vi "LSMcontroller_v65_updatedsealtest.vi"() -> ()   [LabVIEW 2015] (continued)
                    n3079 = property on="save\ndata" class="Bool (strict)"("Value"=TRUE ("save\ndata")) -> ()  [unwired: 2 in, 2 out]
                    n3080 = property on="# of frames" class="DigNum (strict)"("DisabledEnum"=T7."Enabled" ("Disabled")) -> ()  [unwired: 2 in, 2 out]
                  }
                }
              }
              frame #1 {
                n3081 = local read "finite samples"() -> (w6307:bool)
                n3082 = local read "continuous"() -> (w6306:bool)
                n3083 = local read "wavdet"() -> (w6305:bool)
                n3084 = call "2pparameters.vi"("command"="get") -> ("params out"=w6301:T10)  [unwired: 1 in]
                n3085 = Bundle By Name(cluster=w6301, "finite"=w6307, "cont"=w6306, "wavdet"=w6305) -> (w6304:T10)
                n3086 = call "2pparameters.vi"("Params in"=w6304, "command"="set") -> ()  [unwired: 1 out]
              }
            }
          }
          event "continuous": Value Change {
            n3087 = event-data() -> ("NewVal"=w6308:bool)  [unwired: 1 in]
            n3088 = flat-sequence {
              tunnel: w6308 -> [w6309]
              frame #0 {
                n3089 = case shown="True" w6309 {
                  frame False {
                    n3090 = property on="finite samples" class="Bool (strict)"("Value"=TRUE ("finite samples for recording")) -> ()  [unwired: 2 in, 2 out]
                    n3091 = property on="save\ndata" class="Bool (strict)"("Value"=TRUE ("save\ndata")) -> ()  [unwired: 2 in, 2 out]
                    n3092 = property on="wavdet" class="Bool (strict)"("Value"=FALSE ("wavdet")) -> ()  [unwired: 2 in, 2 out]
                    n3093 = local write "Save tab"(enum32{"withsave", "withoutsave"}."withsave" ("Save tab")) -> ()
                    n3094 = property on="# of frames" class="DigNum (strict)"("DisabledEnum"=T7."Enabled" ("Disabled")) -> ()  [unwired: 2 in, 2 out]
                    n3095 = property on="save\ndata" class="Bool (strict)"("DisabledEnum"=T7."Enabled" ("Disabled")) -> ()  [unwired: 2 in, 2 out]
                  }
                  frame True {
                    w6316 = FALSE ("finite samples for recording")
                    n3096 = property on="finite samples" class="Bool (strict)"("Value"=w6316) -> ()  [unwired: 2 in, 2 out]
                    n3097 = property on="wavdet" class="Bool (strict)"("Value"=w6316) -> ()  [unwired: 2 in, 2 out]
                    n3098 = property on="save\ndata" class="Bool (strict)"("Value"=w6316) -> ()  [unwired: 2 in, 2 out]
                    n3099 = local write "Save tab"(enum32{"withsave", "withoutsave"}."withsave" ("Save tab")) -> ()
                    n3100 = property on="# of frames" class="DigNum (strict)"("DisabledEnum"=T7."Disabled and Grayed Out" ("Disabled")) -> ()  [unwired: 2 in, 2 out]
                    n3101 = property on="save\ndata" class="Bool (strict)"("DisabledEnum"=T7."Disabled and Grayed Out" ("Disabled")) -> ()  [unwired: 2 in, 2 out]
                  }
                }
              }
              frame #1 {
                n3102 = local read "finite samples"() -> (w6326:bool)
                n3103 = local read "continuous"() -> (w6325:bool)
                n3104 = local read "wavdet"() -> (w6324:bool)
                n3105 = call "2pparameters.vi"("command"="get") -> ("params out"=w6320:T10)  [unwired: 1 in]
                n3106 = Bundle By Name(cluster=w6320, "finite"=w6326, "cont"=w6325, "wavdet"=w6324) -> (w6323:T10)
                n3107 = call "2pparameters.vi"("Params in"=w6323, "command"="set") -> ()  [unwired: 1 out]
              }
            }
          }
          event "wavdet": Value Change {
            n3108 = event-data() -> ("NewVal"=w6327:bool)  [unwired: 1 in]
            n3109 = flat-sequence {
              tunnel: w6327 -> [w6328]
              frame #0 {
                n3110 = case shown="False" w6328 {
                  frame False {
                    n3111 = property on="finite samples" class="Bool (strict)"("Value"=TRUE ("finite samples for recording")) -> ()  [unwired: 2 in, 2 out]
                    n3112 = property on="continuous" class="Bool (strict)"("Value"=FALSE ("continuous")) -> ()  [unwired: 2 in, 2 out]
                    n3113 = local write "Save tab"(enum32{"withsave", "withoutsave"}."withsave" ("Save tab")) -> ()
                    n3114 = property on="save\ndata" class="Bool (strict)"("DisabledEnum"=T7."Enabled" ("Disabled")) -> ()  [unwired: 2 in, 2 out]
                    n3115 = property on="# of frames" class="DigNum (strict)"("DisabledEnum"=T7."Enabled" ("Disabled")) -> ()  [unwired: 2 in, 2 out]
                    n3116 = property on="save\ndata" class="Bool (strict)"("Value"=TRUE ("save\ndata")) -> ()  [unwired: 2 in, 2 out]
                  }
                  frame True {
                    w6337 = FALSE ("finite samples for recording")
                    n3117 = property on="finite samples" class="Bool (strict)"("Value"=w6337) -> ()  [unwired: 2 in, 2 out]
                    n3118 = property on="continuous" class="Bool (strict)"("Value"=w6337) -> ()  [unwired: 2 in, 2 out]
                    n3119 = property on="save\ndata" class="Bool (strict)"("DisabledEnum"=T7."Enabled" ("Disabled")) -> ()  [unwired: 2 in, 2 out]
                    n3120 = local write "Save tab"(enum32{"withsave", "withoutsave"}."withsave" ("Save tab")) -> ()
                    n3121 = property on="# of frames" class="DigNum (strict)"("DisabledEnum"=T7."Disabled" ("Disabled")) -> ()  [unwired: 2 in, 2 out]
                    n3122 = property on="save\ndata" class="Bool (strict)"("Value"=TRUE ("save\ndata")) -> ()  [unwired: 2 in, 2 out]
                  }
                }
              }
              frame #1 {
                n3123 = local read "finite samples"() -> (w6340:bool)
                n3124 = local read "continuous"() -> (w6341:bool)
                n3125 = local read "wavdet"() -> (w6342:bool)
                n3126 = call "2pparameters.vi"("command"="get") -> ("params out"=w6346:T10)  [unwired: 1 in]
                n3127 = Bundle By Name(cluster=w6346, "finite"=w6340, "cont"=w6341, "wavdet"=w6342) -> (w6343:T10)
                n3128 = call "2pparameters.vi"("Params in"=w6343, "command"="set") -> ()  [unwired: 1 out]
              }
            }
          }
          event "cursors": Value Change {
            n3129 = event-data() -> ()  [unwired: 1 in, 5 out]
            n3130 = case shown="True" "cursors" {
              frame False {
                n3131 = property on="img_CH1" class="IntGraph (strict)"("Active Cursor"=u32 0, "Cursor.Cursor Style"=u8 0 ("Cursor Style"), "Cursor.Cursor Point Style"=u8 0 ("Cursor Point Style")) -> ("Cursor.Cursor Position:Cursor X"=w6351:dbl, "Cursor.Cursor Position:Cursor Y"=w6352:dbl)  [unwired: 2 in, 2 out]
                n3132 = property on="img_CH2" class="IntGraph (strict)"("Active Cursor"=u32 0, "Cursor.Cursor Style"=u8 0 ("Cursor Style"), "Cursor.Cursor Point Style"=u8 0 ("Cursor Point Style")) -> ()  [unwired: 2 in, 2 out]
                n3133 = local write "cursor x [pixel]"(w6351) -> ()
                n3134 = local write "cursor y [pixel]"(w6352) -> ()
              }
              frame True {
                n3135 = stacked-sequence {
                  frame #0 {
                    n3136 = call "2pparameters.vi"("command"="get") -> ("params out"=w6367:T10)  [unwired: 1 in]
                    n3137 = Unbundle By Name(w6367) -> ("Xpixels Img"=w6368:i32, "Ypixels Img"=w6365:i32)
                    n3138 = To Double Precision Float(number=w6365) -> (double precision float=w6359:dbl)
                    n3139 = To Double Precision Float(number=w6368) -> (double precision float=w6364:dbl)
                    n3140 = Divide(x=w6359, y=2.0) -> (x/y=w6360:dbl)
                    n3141 = Divide(x=w6364, y=2.0) -> (x/y=w6362:dbl)
                    n3142 = Round To Nearest(number=w6360) -> (nearest integer value=w6358:dbl)
                    n3143 = Round To Nearest(number=w6362) -> (nearest integer value=w6361:dbl)
                    n3144 = property on="img_CH1" class="IntGraph (strict)"("Active Cursor"=u32 0, "Cursor.Cursor Style"=u8 8 ("Cursor Style"), "Cursor.Cursor Point Style"=u8 5 ("Cursor Point Style"), "Cursor.Cursor Position:Cursor X"=w6361, "Cursor.Cursor Position:Cursor Y"=w6358, "Cursor.Visible"=TRUE) -> ()  [unwired: 2 in, 2 out]
                  }
                  frame #1 {
                    n3145 = call "2pparameters.vi"("command"="get") -> ("params out"=w6387:T10)  [unwired: 1 in]
                    n3146 = call "2pparameters.vi"("command"="get") -> ("params out"=w6385:T10)  [unwired: 1 in]
                    n3147 = property on="img_CH1" class="IntGraph (strict)"("Active Cursor"=u32 0, "Cursor.Cursor Style"=u8 8 ("Cursor Style"), "Cursor.Cursor Point Style"=u8 5 ("Cursor Point Style")) -> ("Cursor.Cursor Position:Cursor X"=w6380:dbl, "Cursor.Cursor Position:Cursor Y"=w6379:dbl, "Cursor.Cursor Index"=w6402:i32, "Cursor.Cursor Plot"=w6401:i32, "Cursor.Visible"=w6372:bool)  [unwired: 2 in, 2 out]
                    "cursor x [pixel]" <- w6380
                    "cursor y [pixel]" <- w6379
                    n3148 = Unbundle By Name(w6387) -> ("Vy-max Img"=w6389:dbl, "Vy-min Img"=w6376:dbl, "Ypixels Img"=w6391:i32)
                    n3149 = Unbundle By Name(w6385) -> ("VX-max Img"=w6386:dbl, "Vx-min Img"=w6374:dbl, "Xpixels Img"=w6390:i32)
                    n3150 = Subtract(x=w6389, y=w6376) -> (x-y=w6394:dbl)
                    n3151 = Subtract(x=w6386, y=w6374) -> (x-y=w6392:dbl)
                    n3152 = local read "img_CH2"() -> (w6398:sgl[][])
                    n3153 = To Double Precision Float(number=w6390) -> (double precision float=w6393:dbl)
                    n3154 = local read "img_CH1"() -> (w6399:sgl[][])
                    n3155 = To Double Precision Float(number=w6391) -> (double precision float=w6395:dbl)
                    n3156 = Index Array(array=w6399, index (row)=w6402, index (col)=w6401) -> (element=→"value CH 1":sgl)
                    n3157 = Index Array(array=w6398, index (row)=w6402, index (col)=w6401) -> (element=→"value CH 2":sgl)
                    n3158 = Divide(x=w6392, y=w6393) -> (x/y=w6396:dbl)
                    n3159 = Divide(x=w6394, y=w6395) -> (x/y=w6397:dbl)
                    n3160 = Multiply(x=w6380, y=w6396) -> (x*y=w6375:dbl)
                    n3161 = Multiply(x=w6379, y=w6397) -> (x*y=w6378:dbl)
                    n3162 = property on="img_CH2" class="IntGraph (strict)"("Active Cursor"=u32 0, "Cursor.Cursor Style"=u8 8 ("Cursor Style"), "Cursor.Cursor Point Style"=u8 5 ("Cursor Point Style"), "Cursor.Cursor Position:Cursor X"=w6380, "Cursor.Cursor Position:Cursor Y"=w6379, "Cursor.Visible"=w6372) -> ()  [unwired: 2 in, 2 out]
                    n3163 = Add(x=w6375, y=w6374) -> (x+y=w6373:dbl)
                    n3164 = Add(x=w6378, y=w6376) -> (x+y=w6377:dbl)
                    n3165 = local write "Vx-ref"(w6373) -> ()
                    n3166 = local write "Vy-ref"(w6377) -> ()
                  }
                }
              }
            }
          }
          event "img_CH1": Cursor Move {
            n3167 = event-data() -> ("CursIdx"=w6407:i32)  [unwired: 1 in]
            n3168 = Equal To 0?(x=w6407) -> (x = 0?=w6408:bool)
            n3169 = case shown="True" w6408 {
              frame False {
              }
              frame True {
                n3170 = call "2pparameters.vi"("command"="get") -> ("params out"=w6428:T10)  [unwired: 1 in]
                n3171 = call "2pparameters.vi"("command"="get") -> ("params out"=w6430:T10)  [unwired: 1 in]
                n3172 = property on="img_CH1" class="IntGraph (strict)"("Active Cursor"=u32 0, "Cursor.Cursor Style"=u8 8 ("Cursor Style"), "Cursor.Cursor Point Style"=u8 5 ("Cursor Point Style")) -> ("Cursor.Cursor Position:Cursor X"=w6417:dbl, "Cursor.Cursor Position:Cursor Y"=w6416:dbl, "Cursor.Cursor Plot"=w6436:i32, "Cursor.Cursor Index"=w6435:i32, "Cursor.Visible"=w6409:bool)  [unwired: 2 in, 2 out]
                n3173 = Unbundle By Name(w6428) -> ("Vy-max Img"=w6426:dbl, "Vy-min Img"=w6415:dbl, "Ypixels Img"=w6424:i32)
                n3174 = Unbundle By Name(w6430) -> ("VX-max Img"=w6429:dbl, "Vx-min Img"=w6410:dbl, "Xpixels Img"=w6425:i32)
                n3175 = Subtract(x=w6426, y=w6415) -> (x-y=w6421:dbl)
                n3176 = Subtract(x=w6429, y=w6410) -> (x-y=w6423:dbl)
                n3177 = local write "cursor x [pixel]"(w6417) -> ()
                n3178 = local write "cursor y [pixel]"(w6416) -> ()
                n3179 = To Double Precision Float(number=w6425) -> (double precision float=w6422:dbl)
                n3180 = To Double Precision Float(number=w6424) -> (double precision float=w6420:dbl)
                n3181 = local read "img_CH2"() -> (w6437:sgl[][])
                n3182 = local read "img_CH1"() -> (w6440:sgl[][])
                n3183 = Index Array(array=w6437, index (row)=w6436, index (col)=w6435) -> (element=w6438:sgl)
                n3184 = Index Array(array=w6440, index (row)=w6436, index (col)=w6435) -> (element=w6439:sgl)
                n3185 = Divide(x=w6423, y=w6422) -> (x/y=w6419:dbl)
                n3186 = Divide(x=w6421, y=w6420) -> (x/y=w6418:dbl)
                n3187 = local write "value CH 2"(w6438) -> ()
                n3188 = Multiply(x=w6417, y=w6419) -> (x*y=w6412:dbl)
                n3189 = local write "value CH 1"(w6439) -> ()
                n3190 = Multiply(x=w6416, y=w6418) -> (x*y=w6414:dbl)
                n3191 = Add(x=w6412, y=w6410) -> (x+y=w6411:dbl)
                n3192 = local write "Vx-ref"(w6411) -> ()
                n3193 = Add(x=w6414, y=w6415) -> (x+y=w6413:dbl)
                n3194 = property on="img_CH2" class="IntGraph (strict)"("Active Cursor"=u32 0, "Cursor.Cursor Style"=u8 8 ("Cursor Style"), "Cursor.Cursor Point Style"=u8 5 ("Cursor Point Style"), "Cursor.Cursor Position:Cursor X"=w6417, "Cursor.Cursor Position:Cursor Y"=w6416, "Cursor.Visible"=w6409) -> ()  [unwired: 2 in, 2 out]
                n3195 = local write "Vy-ref"(w6413) -> ()
              }
            }
          }
          event "img_CH2": Cursor Move {
            n3196 = event-data() -> ("CursIdx"=w6444:i32)  [unwired: 1 in]
            n3197 = Equal To 0?(x=w6444) -> (x = 0?=w6445:bool)
            n3198 = case shown="True" w6445 {
              frame False {
              }
              frame True {
                n3199 = property on="img_CH2" class="IntGraph (strict)"("Active Cursor"=u32 0, "Cursor.Cursor Style"=u8 8 ("Cursor Style"), "Cursor.Cursor Point Style"=u8 5 ("Cursor Point Style")) -> ("Cursor.Cursor Position:Cursor X"=w6453:dbl, "Cursor.Cursor Position:Cursor Y"=w6454:dbl, "Cursor.Cursor Plot"=w6473:i32, "Cursor.Cursor Index"=w6472:i32, "Cursor.Visible"=w6446:bool)  [unwired: 2 in, 2 out]
                n3200 = call "2pparameters.vi"("command"="get") -> ("params out"=w6465:T10)  [unwired: 1 in]
                n3201 = call "2pparameters.vi"("command"="get") -> ("params out"=w6467:T10)  [unwired: 1 in]
                n3202 = local read "img_CH1"() -> (w6477:sgl[][])
                n3203 = local read "img_CH2"() -> (w6474:sgl[][])
                n3204 = local write "cursor x [pixel]"(w6453) -> ()
                n3205 = local write "cursor y [pixel]"(w6454) -> ()
                n3206 = Unbundle By Name(w6465) -> ("Vy-max Img"=w6463:dbl, "Vy-min Img"=w6448:dbl, "Ypixels Img"=w6461:i32)
                n3207 = Unbundle By Name(w6467) -> ("VX-max Img"=w6466:dbl, "Vx-min Img"=w6451:dbl, "Xpixels Img"=w6462:i32)
                n3208 = Index Array(array=w6477, index (row)=w6473, index (col)=w6472) -> (element=w6476:sgl)
                n3209 = Index Array(array=w6474, index (row)=w6473, index (col)=w6472) -> (element=w6475:sgl)
                n3210 = local write "value CH 2"(w6475) -> ()
                n3211 = local write "value CH 1"(w6476) -> ()
                n3212 = Subtract(x=w6463, y=w6448) -> (x-y=w6458:dbl)
                n3213 = Subtract(x=w6466, y=w6451) -> (x-y=w6460:dbl)
                n3214 = To Double Precision Float(number=w6462) -> (double precision float=w6459:dbl)
                n3215 = To Double Precision Float(number=w6461) -> (double precision float=w6457:dbl)
                n3216 = Divide(x=w6460, y=w6459) -> (x/y=w6456:dbl)
                n3217 = Divide(x=w6458, y=w6457) -> (x/y=w6455:dbl)
                n3218 = Multiply(x=w6453, y=w6456) -> (x*y=w6452:dbl)
                n3219 = Multiply(x=w6454, y=w6455) -> (x*y=w6449:dbl)
                n3220 = property on="img_CH1" class="IntGraph (strict)"("Active Cursor"=u32 0, "Cursor.Cursor Style"=u8 8 ("Cursor Style"), "Cursor.Cursor Point Style"=u8 5 ("Cursor Point Style"), "Cursor.Cursor Position:Cursor X"=w6453, "Cursor.Cursor Position:Cursor Y"=w6454, "Cursor.Visible"=w6446) -> ()  [unwired: 2 in, 2 out]
                n3221 = Add(x=w6452, y=w6451) -> (x+y=→"Vx-ref":dbl)
                n3222 = Add(x=w6449, y=w6448) -> (x+y=→"Vy-ref":dbl)
              }
            }
          }
          event "Focus": Value Change {
            n3223 = event-data() -> ()  [unwired: 1 in, 6 out]
            n3224 = flat-sequence {
              frame #0 {
                n3225 = local read "Focus"() -> (w6481:bool)
                n3226 = case shown="True" w6481 {
                  frame False {
                  }
                  frame True {
                    n3227 = local read "Vx-ref"() -> (w6485:dbl)
                    n3228 = local read "Vy-ref"() -> (w6484:dbl)
                    n3229 = local read "zV"() -> (w6482:dbl)
                    n3230 = call "focusvi.vi"("zc"=w6482, "yc"=w6484, "xc"=w6485) -> ("finalz"=→"zV":dbl)
                  }
                }
              }
              frame #1 {
                n3231 = local write "Focus"(FALSE ("Focus")) -> ()
              }
            }
          }
          event "auto shutter": Value Change {
            n3232 = event-data() -> ()  [unwired: 1 in, 6 out]
            n3233 = call "2pparameters.vi"("command"="get") -> ("params out"=w6489:T10)  [unwired: 1 in]
            n3234 = in-place {
              n3235 = in-place-cluster #46(w6489) -> ()  [unwired: 1 out]
              n3236 = local read "auto shutter"() -> (w6491:bool)
              n3237 = in-place-cluster #46("autoshutter"=w6491) -> (w6487:T10)
            }
            n3238 = call "2pparameters.vi"("Params in"=w6487, "command"="set") -> ()  [unwired: 1 out]
          }
          event "auto OD": Value Change {
            n3239 = event-data() -> ()  [unwired: 1 in, 6 out]
            n3240 = call "2pparameters.vi"("command"="get") -> ("params out"=w6494:T10)  [unwired: 1 in]
            n3241 = in-place {
              n3242 = in-place-cluster #47(w6494) -> ()  [unwired: 1 out]
              n3243 = local read "auto OD"() -> (w6496:bool)
              n3244 = in-place-cluster #47("auto OD"=w6496) -> (w6492:T10)
            }
            n3245 = call "2pparameters.vi"("Params in"=w6492, "command"="set") -> ()  [unwired: 1 out]
          }
          event "ODfilt": Value Change {
            n3246 = event-data() -> ("OldVal"=w6497:u16)  [unwired: 1 in, 5 out]
            n3247 = local read "ODfilt"() -> (w6498:u16)
            n3248 = call "2pparameters.vi"("command"="get") -> ("params out"=w6501:T10)  [unwired: 1 in]
            n3249 = call "filterwheelcontrol_nothorlabslib.vi"("Current OD filt"=w6497, "New ODfilt"=w6498) -> ()  [unwired: 1 in]
            n3250 = in-place {
              in-place-border: w6498 -> [w6503]
              n3251 = in-place-cluster #48(w6501) -> ()  [unwired: 1 out]
              n3252 = in-place-cluster #48("ODfilt"=w6503) -> (w6499:T10)
            }
            n3253 = call "2pparameters.vi"("Params in"=w6499, "command"="set") -> ()  [unwired: 1 out]
          }
          event "Exit": Value Change {
            n3254 = event-data() -> ()  [unwired: 1 in, 5 out]
          }
        }
        n3255 = Wait (ms)(milliseconds to wait=u32 50) -> ()  [unwired: 1 out]
      }
      n3256 = while {
        stop <- w69 stop-if-true
        # "Waveform generation"
        n3257 = event shown="[11] \"Load Matlab Waveform\": Value Change" {
          selector: _ -> [_ _ _ _ _ _ _ _ _ _ _ _ _ _ _ _ _ _ _ _ _ _]
          dyn-events: _ -> [_ _ _ _ _ _ _ _ _ _ _ _ _ _ _ _ _ _ _ _ _ _]
          timeout: _ -> [_ _ _ _ _ _ _ _ _ _ _ _ _ _ _ _ _ _ _ _ _ _]
          tunnel: [_ _ _ _ _ _ _ _ _ _ _ _ _ _ _ _ _ _ _ _ _ w2081] -> w69
          event Timeout {
            n3258 = event-data() -> ()  [unwired: 1 in, 3 out]
          }
          event "Add AO wave": Value Change {
            n3259 = event-data() -> ("NewVal"=w70:bool)  [unwired: 1 in, 5 out]
            n3260 = case shown="True" w70 {
              frame False {
              }
              frame True {
                n3261 = stacked-sequence {
                  frame #0 {
                    n3262 = local read "Measurement"() -> (w71:T4)
                    n3263 = case shown="\"Lifetime (contour)\"" w71 {
                      frame "X-Y-t movie", Default {
                        n3264 = local read "avpp"() -> (w92:i32)
                        n3265 = local read "Angle ref"() -> (w91:dbl)
                        n3266 = local read "ROI Type"() -> (w90:u16)
                        n3267 = local read "xpixels ref"() -> (w87:i32)
                        n3268 = local read "Vx-min ref"() -> (w86:dbl)
                        n3269 = local read "Vx-max ref"() -> (w85:dbl)
                        n3270 = local read "ypixels ref"() -> (w83:i32)
                        n3271 = local read "Vy-min ref"() -> (w84:dbl)
                        n3272 = local read "Vy-max ref"() -> (w80:dbl)
                        n3273 = local read "Sampling rate"() -> (w74:dbl)
                        n3274 = local read "finite samples"() -> (w75:bool)
                        n3275 = local read "continuous"() -> (w78:bool)
                        n3276 = local read "wavdet"() -> (w79:bool)
                        n3277 = local read "# of frames"() -> (w77:i32)
                        n3278 = local read "maxbufferAI"() -> (w76:i32)
                        n3279 = local read "Override AI buffer"() -> (w72:bool)
                        n3280 = call "2pparameters.vi"("command"="get") -> ("params out"=w89:T10)  [unwired: 1 in]
                        n3281 = Bundle By Name(cluster=w89, "type"="X-Y-t movie", "avpp"=w92, "Angle Img"=w91, "Xpixels Img"=w87, "Vx-min Img"=w86, "VX-max Img"=w85, "Ypixels Img"=w83, "Vy-min Img"=w84, "Vy-max Img"=w80, "srate"=w74, "srate Img"=w74, "finite"=w75, "cont"=w78, "wavdet"=w79, "measpoints"=w77, "maxbufferAI"=w76, "Drawing Mode"=w90, "Vz-reset"=0.0, "AIoverride"=w72) -> (w81:T10)
                        n3282 = call "2pparameters.vi"("Params in"=w81, "command"="set") -> ()  [unwired: 1 out]
                      }
                      frame "X-Y-Z stack" {
                        n3283 = call "2pparameters.vi"("command"="get") -> ("params out"=w96:T10)  [unwired: 1 in]
                        n3284 = Bundle By Name(cluster=w96, "type"="X-Y-Z stack") -> (w94:T10)
                        n3285 = call "2pparameters.vi"("Params in"=w94, "command"="set") -> ()  [unwired: 1 out]
                      }
                      frame "Lifetime (scan)" {
                        n3286 = call "2pparameters.vi"("command"="get") -> ("params out"=w101:T10)  [unwired: 1 in]
                        n3287 = Bundle By Name(cluster=w101, "type"="Lifetime (scan)") -> (w99:T10)
                        n3288 = call "2pparameters.vi"("Params in"=w99, "command"="set") -> ()  [unwired: 1 out]
                      }
                      frame "Lifetime (contour)" {
                        n3289 = local read "Vy-min draw"() -> (w111:dbl)
                        n3290 = local read "Vy-max draw"() -> (w110:dbl)
                        n3291 = local read "Vx-min draw"() -> (w113:dbl)
                        n3292 = local read "Vx-max draw"() -> (w112:dbl)
                        n3293 = local read "xpixels ref"() -> (w109:i32)
                        n3294 = local read "ypixels ref"() -> (w108:i32)
                        n3295 = local read "ROI Type"() -> (w107:u16)
                        n3296 = local read "srateAODOtt"() -> (w118:dbl)
                        n3297 = local read "# of frames"() -> (w123:i32)
                        n3298 = local read "refreshtime"() -> (w115:dbl)
                        n3299 = local read "Pel"() -> (w106:dbl)
                        n3300 = local read "bin"() -> (w121:dbl)
                        n3301 = local read "Override AI buffer"() -> (w104:bool)
                        n3302 = local read "finite samples"() -> (w130:bool)
                        n3303 = local read "srateAODOtt"() -> (w117:dbl)
                        n3304 = local read "srateAODOtt"() -> (w124:dbl)
                        n3305 = local read "continuous"() -> (w129:bool)
                        n3306 = local read "Angle ref"() -> (w114:dbl)
                        n3307 = local read "wavdet"() -> (w131:bool)
                        n3308 = local read "Vx-ref"() -> (w126:dbl)
                        n3309 = local read "Vy-ref"() -> (w128:dbl)
                        n3310 = local read "avpp"() -> (w127:i32)
                        n3311 = call "tt_timeandsamples.vi"("bin"=w121, "refreshtime"=w115, "srateAODOtt"=w118, "tot#ofsamples"=w123) -> ("refreshrate"=w119:dbl, "refreshbuffer"=w120:i32, "timetracecycles"=w125:i32)  [unwired: 5 in]
                        n3312 = local read "bin"() -> (w122:dbl)
                        n3313 = call "2pparameters.vi"("command"="get") -> ("params out"=w134:T10)  [unwired: 1 in]
                        n3314 = Bundle By Name(cluster=w134, "Drawing Mode"=w107, "measpoints"=w123, "tt_cycles"=w125, "refreshbuffer"=w120, "refreshrate"=w119, "Vx-ref"=w126, "Vy-ref"=w128, "srate"=w117, "finite"=w130, "cont"=w129, "wavdet"=w131, "avpp"=w127, "srateAODO"=w124, "bufferAI"=w120, "bin"=w122, "Angle Img"=w114, "Vxminref"=w113, "Vxmaxref"=w112, "Vyminref"=w111, "Vymaxref"=w110, "Xpixels Img"=w109, "Ypixels Img"=w108, "Pel"=w106, "Vz-reset"=0.0, "AIoverride"=w104, "type"="Lifetime (contour)") -> (w132:T10)
                        n3315 = Reciprocal(x=w119) -> (1/x=w116:dbl)
                        n3316 = local write "refreshtime"(w116) -> ()
                        n3317 = call "2pparameters.vi"("Params in"=w132, "command"="set") -> ()  [unwired: 1 out]
                      }
                      frame "X-Y-Z-t movie" {
                      }
                      frame "linescan" {
                      }
                      frame "Timetrace" {
                        n3318 = local read "Vy-min draw"() -> (w144:dbl)
                        n3319 = local read "Vy-max draw"() -> (w143:dbl)
                        n3320 = local read "Vx-min draw"() -> (w146:dbl)
                        n3321 = local read "Vx-max draw"() -> (w145:dbl)
                        n3322 = local read "xpixels ref"() -> (w142:i32)
                        n3323 = local read "ypixels ref"() -> (w141:i32)
                        n3324 = local read "ROI Type"() -> (w140:u16)
                        n3325 = local read "srateAODOtt"() -> (w151:dbl)
                        n3326 = local read "# of frames"() -> (w156:i32)
                        n3327 = local read "refreshtime"() -> (w148:dbl)
                        n3328 = local read "Pel"() -> (w139:dbl)
                        n3329 = local read "bin"() -> (w154:dbl)
                        n3330 = local read "Override AI buffer"() -> (w137:bool)
                        n3331 = local read "finite samples"() -> (w163:bool)
                        n3332 = local read "srateAODOtt"() -> (w150:dbl)
                        n3333 = local read "srateAODOtt"() -> (w157:dbl)
                        n3334 = local read "continuous"() -> (w162:bool)
                        n3335 = local read "Angle ref"() -> (w147:dbl)
                        n3336 = local read "wavdet"() -> (w164:bool)
                        n3337 = local read "Vx-ref"() -> (w159:dbl)
                        n3338 = local read "Vy-ref"() -> (w161:dbl)
                        n3339 = local read "avpp"() -> (w160:i32)
                        n3340 = call "tt_timeandsamples.vi"("bin"=w154, "refreshtime"=w148, "srateAODOtt"=w151, "tot#ofsamples"=w156) -> ("refreshrate"=w152:dbl, "refreshbuffer"=w153:i32, "timetracecycles"=w158:i32)  [unwired: 5 in]
                        n3341 = local read "bin"() -> (w155:dbl)
                        n3342 = call "2pparameters.vi"("command"="get") -> ("params out"=w167:T10)  [unwired: 1 in]
                        n3343 = Bundle By Name(cluster=w167, "Drawing Mode"=w140, "measpoints"=w156, "tt_cycles"=w158, "refreshbuffer"=w153, "refreshrate"=w152, "Vx-ref"=w159, "Vy-ref"=w161, "srate"=w150, "finite"=w163, "cont"=w162, "wavdet"=w164, "avpp"=w160, "srateAODO"=w157, "bufferAI"=w153, "bin"=w155, "Angle Img"=w147, "Vxminref"=w146, "Vxmaxref"=w145, "Vyminref"=w144, "Vymaxref"=w143, "Xpixels Img"=w142, "Ypixels Img"=w141, "Pel"=w139, "Vz-reset"=0.0, "AIoverride"=w137, "type"="Timetrace") -> (w165:T10)
                        n3344 = Reciprocal(x=w152) -> (1/x=w149:dbl)
                        n3345 = local write "refreshtime"(w149) -> ()
                        n3346 = call "2pparameters.vi"("Params in"=w165, "command"="set") -> ()  [unwired: 1 out]
                      }
                      frame "Lifetime (point)" {
                      }
                    }
                  }
                  frame #1 {
                    w170 = FALSE ("wavdet")
                    n3347 = call "2pparameters.vi"("command"="get") -> ("params out"=w174:T10)  [unwired: 1 in]
                    n3348 = Bundle By Name(cluster=w174, "finite"=w170, "cont"=w170, "wavdet"=TRUE) -> (w171:T10)
                    n3349 = call "2pparameters.vi"("Params in"=w171, "command"="set") -> ()  [unwired: 1 out]
                  }
                  frame #2 {
                    # "change active waveform numbers array"
                    n3350 = local read "AO channels"() -> (w181:u32)
                    n3351 = call "2pparameters.vi"("command"="get") -> ("params out"=w179:T10)  [unwired: 1 in]
                    n3352 = in-place {
                      in-place-border: w181 -> [w185]
                      in-place-border: [w182] -> w176
                      n3353 = in-place-cluster #49(w179) -> ("aAO"=w184:u32[])
                      n3354 = call "add channel to active arrayv2.vi"("line array in"=w184, "line to add"=w185) -> ("line array out"=w183:u32[], "addition"=w182:bool)  [unwired: 1 out]
                      n3355 = in-place-cluster #49("aAO"=w183) -> (w177:T10)
                    }
                    n3356 = local write "addAO"(w176) -> ()
                    n3357 = call "2pparameters.vi"("Params in"=w177, "command"="set") -> ()  [unwired: 1 out]
                  }
                  frame #3 {
                    # "update GUI"
                    n3358 = local read "addAO"() -> (w186:bool)
                    n3359 = case shown="True" w186 {
                      frame False {
                      }
                      frame True {
                        n3360 = call "Used AO lines.vi"() -> ("used AO names"=w190:string[], "used AO lines"=w192:tag[])  [unwired: 2 in]
                        n3361 = control-ref of="Analog Lines Plot"() -> (w191:refnum<vi>)
                        n3362 = control-ref of="Digital Lines Plot"() -> (w189:refnum<vi>)
                        n3363 = call "Used DO lines.vi"() -> ("used DO names"=w188:string[], "used DO lines"=w187:tag[])  [unwired: 2 in]
                        n3364 = local write "Analog Used Lines"(w192) -> ()
                        n3365 = local write "Analog Used Names"(w190) -> ()
                        n3366 = local write "Digital Used Lines"(w187) -> ()
                        n3367 = local write "Digital Used Names"(w188) -> ()
                        n3368 = call "prepDOWaveplot.vi"("DigitalGraph in"=w189, "used DO names"=w188) -> ()  [unwired: 1 in]
                        n3369 = call "prepAOWaveplot.vi"("WaveformGraph in"=w191, "Analog Used Names"=w190) -> ()  [unwired: 1 in]
                      }
                    }
                  }
                  frame #4 {
                    n3370 = local read "addAO"() -> (w193:bool)
                    n3371 = case shown="True" w193 {
                      frame False {
                      }
                      frame True {
                        # "add parameters\nto parameter array"
                        n3372 = local read "Build analog waveform tabs"() -> (w194:enum32{"Square", "Triangle", "Matlab"})
                        n3373 = case shown="\"Matlab\"" w194 {
                          frame "Square", Default {
                            w207 = 0.0 ("Offset (V)")
                            n3374 = local read "Meastab"() -> (w196:enum32{"X-Y Image", "Linescan", "Timetrace"})
                            n3375 = call "waveformparamsv2.vi"("command"="get") -> ("Params out"=w205:T14)  [unwired: 4 in, 2 out]
                            n3376 = Unbundle By Name(w205) -> ("AO parameters"=w202:T15)
                            n3377 = case shown="\"Timetrace\"" w196 {
                              tunnel: [w218 w219] -> w195
                              frame "X-Y Image", Default {
                                n3378 = local read "Sampling rate"() -> (w218:dbl)
                              }
                              frame "Timetrace" {
                                n3379 = local read "srateAODOtt"() -> (w219:dbl)
                              }
                            }
                            n3380 = local read "Start amplitude (V)"() -> (w215:dbl)
                            n3381 = local read "phase shift (ms)"() -> (w208:dbl)
                            n3382 = local read "Step size (V)"() -> (w213:dbl)
                            n3383 = local read "Baseline (V)"() -> (w214:dbl)
                            n3384 = local read "Period (ms)"() -> (w211:dbl)
                            n3385 = local read "padding value"() -> (w198:dbl)
                            n3386 = local read "Repeats"() -> (w217:dbl)
                            n3387 = local read "DC (%)"() -> (w212:dbl)
                            n3388 = local read "Cycles"() -> (w216:dbl)
                            n3389 = local read "Pulses"() -> (w209:dbl)
                            n3390 = Index Array(array=w202, index=0) -> (element=w203:T16)
                            n3391 = Bundle By Name(cluster=w203, "AOtab"=0.0 ("Repeats"), "Repeats"=w217, "Cycles"=w216, "Start amplitude (V)"=w215, "Baseline (V)"=w214, "Step size (V)"=w213, "DC (%)"=w212, "Sampling frequency (Hz)"=w195, "Period (ms)"=w211, "Offset (V)"=w207, "Amplitude (V)"=w207, "Frequency"=w207, "Tri Repeats"=w207, "phase shift (ms)"=w208, "Pulses"=w209, "Matlab wave file"=path "", "padding value"=w198) -> (w200:T16)
                            n3392 = Build Array(w200) -> (w199:T15)
                            n3393 = call "waveformparamsv2.vi"("command"="add AO", "add AO"=w199) -> ()  [unwired: 3 in, 3 out]
                          }
                          frame "Matlab" {
                            w225 = 0.0 ("Repeats")
                            n3394 = local read "Meastab"() -> (w221:enum32{"X-Y Image", "Linescan", "Timetrace"})
                            n3395 = call "waveformparamsv2.vi"("command"="get") -> ("Params out"=w232:T14)  [unwired: 4 in, 2 out]
                            n3396 = Unbundle By Name(w232) -> ("AO parameters"=w229:T15)
                            n3397 = case shown="\"Timetrace\"" w221 {
                              tunnel: [w235 w236] -> w220
                              frame "X-Y Image", Default {
                                n3398 = local read "Sampling rate"() -> (w235:dbl)
                              }
                              frame "Timetrace" {
                                n3399 = local read "srateAODOtt"() -> (w236:dbl)
                              }
                            }
                            n3400 = local read "Matlab waveform path"() -> (w222:path)
                            n3401 = local read "Matlab padding value"() -> (w224:dbl)
                            n3402 = Index Array(array=w229, index=0) -> (element=w230:T16)
                            n3403 = call "matlabwfexistsdialogue.vi"("Matlab waveform path"=w222) -> ("mtalab waveform path out"=w223:path)
                            n3404 = Bundle By Name(cluster=w230, "AOtab"=2.0 ("Repeats"), "Repeats"=w225, "Cycles"=w225, "Start amplitude (V)"=w225, "Baseline (V)"=w225, "Step size (V)"=w225, "DC (%)"=w225, "Sampling frequency (Hz)"=w220, "Period (ms)"=w225, "Offset (V)"=w225, "Amplitude (V)"=w225, "Frequency"=w225, "Tri Repeats"=w225, "phase shift (ms)"=w225, "Pulses"=w225, "Matlab wave file"=w223, "padding value"=w224) -> (w227:T16)
                            n3405 = Build Array(w227) -> (w226:T15)
                            n3406 = call "waveformparamsv2.vi"("command"="add AO", "add AO"=w226) -> ()  [unwired: 3 in, 3 out]
                          }
                          frame "Triangle" {
                            w242 = 0.0 ("Offset (V)")
                            n3407 = local read "Meastab"() -> (w238:enum32{"X-Y Image", "Linescan", "Timetrace"})
                            n3408 = call "waveformparamsv2.vi"("command"="get") -> ("Params out"=w254:T14)  [unwired: 4 in, 2 out]
                            n3409 = Unbundle By Name(w254) -> ("AO parameters"=w251:T15)
                            n3410 = case shown="\"Timetrace\"" w238 {
                              tunnel: [w256 w257] -> w237
                              frame "X-Y Image", Default {
                                n3411 = local read "Sampling rate"() -> (w256:dbl)
                              }
                              frame "Timetrace" {
                                n3412 = local read "srateAODOtt"() -> (w257:dbl)
                              }
                            }
                            n3413 = local read "Tri padding value"() -> (w240:dbl)
                            n3414 = local read "Amplitude (V)"() -> (w245:dbl)
                            n3415 = local read "Tri Phase (s)"() -> (w241:dbl)
                            n3416 = local read "Tri Repeats"() -> (w243:dbl)
                            n3417 = local read "Frequency"() -> (w244:dbl)
                            n3418 = local read "Offset (V)"() -> (w246:dbl)
                            n3419 = Index Array(array=w251, index=0) -> (element=w252:T16)
                            n3420 = Bundle By Name(cluster=w252, "AOtab"=1.0 ("Repeats"), "Repeats"=w242, "Cycles"=w242, "Start amplitude (V)"=w242, "Baseline (V)"=w242, "Step size (V)"=w242, "DC (%)"=w242, "Sampling frequency (Hz)"=w237, "Period (ms)"=w242, "Offset (V)"=w246, "Amplitude (V)"=w245, "Frequency"=w244, "Tri Repeats"=w243, "phase shift (ms)"=w242, "Pulses"=w242, "Matlab wave file"=path "", "Tri phase"=w241, "padding value"=w240) -> (w249:T16)
                            n3421 = Build Array(w249) -> (w248:T15)
                            n3422 = call "waveformparamsv2.vi"("command"="add AO", "add AO"=w248) -> ()  [unwired: 3 in, 3 out]
                          }
                        }
                      }
                    }
                  }
                  frame #5 {
                    n3423 = local read "addAO"() -> (w258:bool)
                    n3424 = case shown="True" w258 {
                      frame False {
                      }
                      frame True {
                        # "add waveform to waveform array; correct waveform lengths and plot"
                        n3425 = local read "Meastab"() -> (w262:enum32{"X-Y Image", "Linescan", "Timetrace"})
                        n3426 = local read "Build analog waveform tabs"() -> (w272:enum32{"Square", "Triangle", "Matlab"})
                        n3427 = case shown="\"Timetrace\"" w262 {
                          tunnel: [w280 w281] -> w261
                          frame "X-Y Image", Default {
                            n3428 = local read "Sampling rate"() -> (w280:dbl)
                          }
                          frame "Timetrace" {
                            n3429 = local read "srateAODOtt"() -> (w281:dbl)
                          }
                        }
                        n3430 = call "waveformparamsv2.vi"("command"="get last AO") -> ("last AO"=w274:T16)  [unwired: 4 in, 2 out]
                        n3431 = case shown="\"Matlab\"" w272 {
                          tunnel: w274 -> [w284 w286 w288]
                          tunnel: [w283 w285 w287] -> w273
                          frame "Square", Default {
                            n3432 = call "generateRampedSquareWave_fromAOparameters.vi"("AO params"=w284) -> ("Waveform"=w283:waveform(dbl))  [unwired: 1 out]
                          }
                          frame "Triangle" {
                            n3433 = call "generateTriWave_fromAOparameters.vi"("AO params"=w286) -> ("Waveform"=w285:waveform(dbl))  [unwired: 1 out]
                          }
                          frame "Matlab" {
                            n3434 = call "matlabAOwffromparam.vi"("Cluster"=w288) -> ("Waveform"=w287:waveform(dbl))  [unwired: 1 out]
                          }
                        }
                        n3435 = property on="refwf" class="Ring (strict)"() -> ("RingText.Text"=w265:string)  [unwired: 2 in, 2 out]
                        n3436 = call "waveformsAObuffer.vi"("command"="get") -> ("AO wf out"=w278:waveform(dbl)[])  [unwired: 1 in]
                        n3437 = Build Array (concatenate)(w278, w273) -> (w275:waveform(dbl)[])
                        n3438 = call "waveformsDObuffer.vi"("command"="get") -> ("DO wf out"=w270:digitalwaveform[])  [unwired: 1 in]
                        n3439 = call "correctwaveformsizetemp.vi"("new sampling frequency (Hz)"=w261, "start"=FALSE, "reference waveforms to"=w265, "Analog waveforms in"=w275, "stop"=FALSE, "Digital waveforms in"=w270) -> ("analog wf out"=w268:waveform(dbl)[], "Digital wf out"=w266:digitalwaveform[], "measpoints"=w263:i32)
                        n3440 = local write "Analog Lines Plot"(w268) -> ()
                        n3441 = call "GetNumCamFramesv2.vi"("Digital Waveform Graph"=w266) -> ("Numeric"=w267:i32)  [unwired: 10 in]
                        n3442 = local write "Digital Lines Plot"(w266) -> ()
                        n3443 = call "waveformsAObuffer.vi"("AO wf in"=w268, "command"="set") -> ()  [unwired: 1 out]
                        n3444 = call "waveformsDObuffer.vi"("DO wf in"=w266, "command"="set") -> ()  [unwired: 1 out]
                        n3445 = local write "Total Camera Frames"(w267) -> ()
                        n3446 = local read "wavdet"() -> (w264:bool)
                        n3447 = case shown="True" w264 {
                          tunnel: w263 -> [_ w282]
                          frame False {
                          }
                          frame True {
                            n3448 = local write "# of frames"(w282) -> ()
                          }
                        }
                      }
                    }
                  }
                  frame #6 {
                    w290 = FALSE ("addAO")
                    # "set signaling boolean to false"
                    n3449 = local read "Build analog waveform tabs"() -> (w289:enum32{"Square", "Triangle", "Matlab"})
                    n3450 = local read "finite samples"() -> (w291:bool)
                    n3451 = local read "continuous"() -> (w292:bool)
                    n3452 = local read "wavdet"() -> (w293:bool)
                    n3453 = call "2pparameters.vi"("command"="get") -> ("params out"=w296:T10)  [unwired: 1 in]
                    n3454 = Bundle By Name(cluster=w296, "finite"=w291, "cont"=w292, "wavdet"=w293) -> (w294:T10)
                    n3455 = case shown="\"Matlab\"" w289 {
                      frame "Square", Default {
                        n3456 = local write "not loaded"(FALSE ("not loaded")) -> ()
                      }
                      frame "Triangle" {
                        n3457 = local write "not loadedtri"(FALSE ("not loadedtri")) -> ()
                      }
                      frame "Matlab" {
                        n3458 = local write "not loadedml"(FALSE ("not loadedml")) -> ()
                      }
                    }
                    n3459 = local write "addAO"(w290) -> ()
                    n3460 = property on="Add AO wave" class="Bool (strict)"("Val(Sgnl)"=w290) -> ()  [unwired: 2 in, 2 out]
                    n3461 = call "2pparameters.vi"("Params in"=w294, "command"="set") -> ()  [unwired: 1 out]
                  }
                }
              }
            }
          }
          event "AO channels": Value Change {
            n3462 = event-data() -> ()  [unwired: 1 in, 6 out]
            n3463 = local read "AO channels"() -> (w301:u32)
            n3464 = call "2pparameters.vi"("command"="get") -> ("params out"=w303:T10)  [unwired: 1 in]
            n3465 = Unbundle By Name(w303) -> ("aAO"=w302:u32[])
            n3466 = Search 1D Array(1D array=w302, element=w301) -> (index of element=w305:i32)  [unwired: 1 in]
            n3467 = Equal?(x=w305, y=-1.0) -> (x = y?=w306:bool)
            n3468 = case shown="False" w306 {
              tunnel: w305 -> [w308 _]
              frame False {
                n3469 = call "waveformparamsv2.vi"("command"="get") -> ("Params out"=w315:T14)  [unwired: 4 in, 2 out]
                n3470 = Unbundle By Name(w315) -> ("AO parameters"=w314:T15)
                n3471 = Index Array(array=w314, index=w308) -> (element=w331:T16)
                n3472 = Unbundle By Name(w331) -> ("AOtab"=w312:dbl, "Repeats"=w330:dbl, "Cycles"=w329:dbl, "Start amplitude (V)"=w328:dbl, "Baseline (V)"=w327:dbl, "Step size (V)"=w326:dbl, "DC (%)"=w325:dbl, "Sampling frequency (Hz)"=w324:dbl, "Period (ms)"=w323:dbl, "Offset (V)"=w322:dbl, "Amplitude (V)"=w321:dbl, "Frequency"=w320:dbl, "Tri Repeats"=w319:dbl, "phase shift (ms)"=w318:dbl, "Pulses"=w317:dbl, "Tri phase"=w313:dbl, "padding value"=w309:dbl, "Matlab wave file"=w310:path)
                n3473 = To Unsigned Long Integer(number=w312) -> (unsigned 32bit integer=w311:u32)
                n3474 = local write "Build analog waveform tabs"(w311) -> ()
                n3475 = local write "Matlab waveform path"(w310) -> ()
                n3476 = local write "phase shift (ms)"(w318) -> ()
                n3477 = local write "Repeats"(w330) -> ()
                n3478 = local write "Cycles"(w329) -> ()
                n3479 = local write "Amplitude (V)"(w321) -> ()
                n3480 = local write "Matlab padding value"(w309) -> ()
                n3481 = local write "Tri padding value"(w309) -> ()
                n3482 = local write "Start amplitude (V)"(w328) -> ()
                n3483 = local write "Tri Phase (s)"(w313) -> ()
                n3484 = local write "Period (ms)"(w323) -> ()
                n3485 = local write "Tri Repeats"(w319) -> ()
                n3486 = local write "Offset (V)"(w322) -> ()
                n3487 = local write "Frequency"(w320) -> ()
                n3488 = local write "Pulses"(w317) -> ()
                n3489 = local write "padding value"(w309) -> ()
                n3490 = local write "Sampling rate \ncurrent wf"(w324) -> ()
                n3491 = local write "Baseline (V)"(w327) -> ()
                n3492 = local write "Step size (V)"(w326) -> ()
                n3493 = local write "DC (%)"(w325) -> ()
              }
              frame True {
              }
            }
          }
          event "Rem AO wave": Value Change {
            n3494 = event-data() -> ("NewVal"=w332:bool)  [unwired: 1 in, 5 out]
            n3495 = case shown="True" w332 {
              frame False {
              }
              frame True {
                n3496 = stacked-sequence {
                  seq-local: [_ _ w438 _ _ _ _] -> [_ _ _ _ w458 w461 _]
                  frame #0 {
                    n3497 = local read "Measurement"() -> (w333:T4)
                    n3498 = case shown="\"X-Y-t movie\", Default" w333 {
                      frame "X-Y-t movie", Default {
                        n3499 = local read "avpp"() -> (w354:i32)
                        n3500 = local read "Angle ref"() -> (w353:dbl)
                        n3501 = local read "ROI Type"() -> (w352:u16)
                        n3502 = local read "xpixels ref"() -> (w349:i32)
                        n3503 = local read "Vx-min ref"() -> (w348:dbl)
                        n3504 = local read "Vx-max ref"() -> (w347:dbl)
                        n3505 = local read "ypixels ref"() -> (w345:i32)
                        n3506 = local read "Vy-min ref"() -> (w346:dbl)
                        n3507 = local read "Vy-max ref"() -> (w342:dbl)
                        n3508 = local read "Sampling rate"() -> (w336:dbl)
                        n3509 = local read "finite samples"() -> (w337:bool)
                        n3510 = local read "continuous"() -> (w340:bool)
                        n3511 = local read "wavdet"() -> (w341:bool)
                        n3512 = local read "# of frames"() -> (w339:i32)
                        n3513 = local read "maxbufferAI"() -> (w338:i32)
                        n3514 = local read "Override AI buffer"() -> (w334:bool)
                        n3515 = call "2pparameters.vi"("command"="get") -> ("params out"=w351:T10)  [unwired: 1 in]
                        n3516 = Bundle By Name(cluster=w351, "type"="X-Y-t movie", "avpp"=w354, "Angle Img"=w353, "Xpixels Img"=w349, "Vx-min Img"=w348, "VX-max Img"=w347, "Ypixels Img"=w345, "Vy-min Img"=w346, "Vy-max Img"=w342, "srate"=w336, "srate Img"=w336, "finite"=w337, "cont"=w340, "wavdet"=w341, "measpoints"=w339, "maxbufferAI"=w338, "Drawing Mode"=w352, "Vz-reset"=0.0, "AIoverride"=w334) -> (w343:T10)
                        n3517 = call "2pparameters.vi"("Params in"=w343, "command"="set") -> ()  [unwired: 1 out]
                      }
                      frame "X-Y-Z stack" {
                        n3518 = call "2pparameters.vi"("command"="get") -> ("params out"=w358:T10)  [unwired: 1 in]
                        n3519 = Bundle By Name(cluster=w358, "type"="X-Y-Z stack") -> (w356:T10)
                        n3520 = call "2pparameters.vi"("Params in"=w356, "command"="set") -> ()  [unwired: 1 out]
                      }
                      frame "Lifetime (scan)" {
                        n3521 = call "2pparameters.vi"("command"="get") -> ("params out"=w363:T10)  [unwired: 1 in]
                        n3522 = Bundle By Name(cluster=w363, "type"="Lifetime (scan)") -> (w361:T10)
                        n3523 = call "2pparameters.vi"("Params in"=w361, "command"="set") -> ()  [unwired: 1 out]
                      }
                      frame "Lifetime (contour)" {
                        n3524 = local read "Vy-min draw"() -> (w373:dbl)
                        n3525 = local read "Vy-max draw"() -> (w372:dbl)
                        n3526 = local read "Vx-min draw"() -> (w375:dbl)
                        n3527 = local read "Vx-max draw"() -> (w374:dbl)
                        n3528 = local read "xpixels ref"() -> (w371:i32)
                        n3529 = local read "ypixels ref"() -> (w370:i32)
                        n3530 = local read "ROI Type"() -> (w369:u16)
                        n3531 = local read "srateAODOtt"() -> (w380:dbl)
                        n3532 = local read "# of frames"() -> (w385:i32)
                        n3533 = local read "refreshtime"() -> (w377:dbl)
                        n3534 = local read "Pel"() -> (w368:dbl)
                        n3535 = local read "bin"() -> (w383:dbl)
                        n3536 = local read "Override AI buffer"() -> (w366:bool)
                        n3537 = local read "finite samples"() -> (w392:bool)
                        n3538 = local read "srateAODOtt"() -> (w379:dbl)
                        n3539 = local read "srateAODOtt"() -> (w386:dbl)
                        n3540 = local read "continuous"() -> (w391:bool)
                        n3541 = local read "Angle ref"() -> (w376:dbl)
                        n3542 = local read "wavdet"() -> (w393:bool)
                        n3543 = local read "Vx-ref"() -> (w388:dbl)
                        n3544 = local read "Vy-ref"() -> (w390:dbl)
                        n3545 = local read "avpp"() -> (w389:i32)
                        n3546 = call "tt_timeandsamples.vi"("bin"=w383, "refreshtime"=w377, "srateAODOtt"=w380, "tot#ofsamples"=w385) -> ("refreshrate"=w381:dbl, "refreshbuffer"=w382:i32, "timetracecycles"=w387:i32)  [unwired: 5 in]
                        n3547 = local read "bin"() -> (w384:dbl)
                        n3548 = call "2pparameters.vi"("command"="get") -> ("params out"=w396:T10)  [unwired: 1 in]
                        n3549 = Bundle By Name(cluster=w396, "Drawing Mode"=w369, "measpoints"=w385, "tt_cycles"=w387, "refreshbuffer"=w382, "refreshrate"=w381, "Vx-ref"=w388, "Vy-ref"=w390, "srate"=w379, "finite"=w392, "cont"=w391, "wavdet"=w393, "avpp"=w389, "srateAODO"=w386, "bufferAI"=w382, "bin"=w384, "Angle Img"=w376, "Vxminref"=w375, "Vxmaxref"=w374, "Vyminref"=w373, "Vymaxref"=w372, "Xpixels Img"=w371, "Ypixels Img"=w370, "Pel"=w368, "Vz-reset"=0.0, "AIoverride"=w366, "type"="Lifetime (contour)") -> (w394:T10)
                        n3550 = Reciprocal(x=w381) -> (1/x=w378:dbl)
                        n3551 = local write "refreshtime"(w378) -> ()
                        n3552 = call "2pparameters.vi"("Params in"=w394, "command"="set") -> ()  [unwired: 1 out]
                      }
                      frame "X-Y-Z-t movie" {
                      }
                      frame "linescan" {
                      }
                      frame "Timetrace" {
                        n3553 = local read "Vy-min draw"() -> (w406:dbl)
                        n3554 = local read "Vy-max draw"() -> (w405:dbl)
                        n3555 = local read "Vx-min draw"() -> (w408:dbl)
                        n3556 = local read "Vx-max draw"() -> (w407:dbl)
                        n3557 = local read "xpixels ref"() -> (w404:i32)
                        n3558 = local read "ypixels ref"() -> (w403:i32)
                        n3559 = local read "ROI Type"() -> (w402:u16)
                        n3560 = local read "srateAODOtt"() -> (w413:dbl)
                        n3561 = local read "# of frames"() -> (w418:i32)
                        n3562 = local read "refreshtime"() -> (w410:dbl)
                        n3563 = local read "Pel"() -> (w401:dbl)
                        n3564 = local read "bin"() -> (w416:dbl)
                        n3565 = local read "Override AI buffer"() -> (w399:bool)
                        n3566 = local read "finite samples"() -> (w425:bool)
                        n3567 = local read "srateAODOtt"() -> (w412:dbl)
                        n3568 = local read "srateAODOtt"() -> (w419:dbl)
                        n3569 = local read "continuous"() -> (w424:bool)
                        n3570 = local read "Angle ref"() -> (w409:dbl)
                        n3571 = local read "wavdet"() -> (w426:bool)
                        n3572 = local read "Vx-ref"() -> (w421:dbl)
                        n3573 = local read "Vy-ref"() -> (w423:dbl)
                        n3574 = local read "avpp"() -> (w422:i32)
                        n3575 = call "tt_timeandsamples.vi"("bin"=w416, "refreshtime"=w410, "srateAODOtt"=w413, "tot#ofsamples"=w418) -> ("refreshrate"=w414:dbl, "refreshbuffer"=w415:i32, "timetracecycles"=w420:i32)  [unwired: 5 in]
                        n3576 = local read "bin"() -> (w417:dbl)
                        n3577 = call "2pparameters.vi"("command"="get") -> ("params out"=w429:T10)  [unwired: 1 in]
                        n3578 = Bundle By Name(cluster=w429, "Drawing Mode"=w402, "measpoints"=w418, "tt_cycles"=w420, "refreshbuffer"=w415, "refreshrate"=w414, "Vx-ref"=w421, "Vy-ref"=w423, "srate"=w412, "finite"=w425, "cont"=w424, "wavdet"=w426, "avpp"=w422, "srateAODO"=w419, "bufferAI"=w415, "bin"=w417, "Angle Img"=w409, "Vxminref"=w408, "Vxmaxref"=w407, "Vyminref"=w406, "Vymaxref"=w405, "Xpixels Img"=w404, "Ypixels Img"=w403, "Pel"=w401, "Vz-reset"=0.0, "AIoverride"=w399, "type"="Timetrace") -> (w427:T10)
                        n3579 = Reciprocal(x=w414) -> (1/x=w411:dbl)
                        n3580 = local write "refreshtime"(w411) -> ()
                        n3581 = call "2pparameters.vi"("Params in"=w427, "command"="set") -> ()  [unwired: 1 out]
                      }
                      frame "Lifetime (point)" {
                      }
                    }
                  }
                  frame #1 {
                    w432 = FALSE ("wavdet")
                    n3582 = call "2pparameters.vi"("command"="get") -> ("params out"=w436:T10)  [unwired: 1 in]
                    n3583 = Bundle By Name(cluster=w436, "finite"=w432, "cont"=w432, "wavdet"=TRUE) -> (w433:T10)
                    n3584 = call "2pparameters.vi"("Params in"=w433, "command"="set") -> ()  [unwired: 1 out]
                  }
                  frame #2 {
                    # "remove channel from numbers array"
                    n3585 = local read "AO channels"() -> (w443:u32)
                    n3586 = call "2pparameters.vi"("command"="get") -> ("params out"=w441:T10)  [unwired: 1 in]
                    n3587 = in-place {
                      in-place-border: w443 -> [w449]
                      in-place-border: [w446] -> w444
                      in-place-border: [w445] -> w438
                      n3588 = in-place-cluster #50(w441) -> ("aAO"=w448:u32[])
                      n3589 = call "remove channel from active arrayv2.vi"("line array in"=w448, "line to remove"=w449) -> ("line array out"=w447:u32[], "removal"=w446:bool, "index"=w445:i32)
                      n3590 = in-place-cluster #50("aAO"=w447) -> (w439:T10)
                    }
                    n3591 = local write "remAO"(w444) -> ()
                    n3592 = call "2pparameters.vi"("Params in"=w439, "command"="set") -> ()  [unwired: 1 out]
                  }
                  frame #3 {
                    n3593 = local read "remAO"() -> (w450:bool)
                    n3594 = case shown="True" w450 {
                      frame False {
                      }
                      frame True {
                        n3595 = call "Used AO lines.vi"() -> ("used AO names"=w454:string[], "used AO lines"=w456:tag[])  [unwired: 2 in]
                        n3596 = control-ref of="Analog Lines Plot"() -> (w455:refnum<vi>)
                        n3597 = control-ref of="Digital Lines Plot"() -> (w453:refnum<vi>)
                        n3598 = call "Used DO lines.vi"() -> ("used DO names"=w452:string[], "used DO lines"=w451:tag[])  [unwired: 2 in]
                        n3599 = local write "Analog Used Lines"(w456) -> ()
                        n3600 = local write "Analog Used Names"(w454) -> ()
                        n3601 = local write "Digital Used Lines"(w451) -> ()
                        n3602 = local write "Digital Used Names"(w452) -> ()
                        n3603 = call "prepDOWaveplot.vi"("DigitalGraph in"=w453, "used DO names"=w452) -> ()  [unwired: 1 in]
                        n3604 = call "prepAOWaveplot.vi"("WaveformGraph in"=w455, "Analog Used Names"=w454) -> ()  [unwired: 1 in]
                      }
                    }
                  }
                  frame #4 {
                    n3605 = local read "remAO"() -> (w457:bool)
                    n3606 = case shown="True" w457 {
                      tunnel: w458 -> [_ w459]
                      frame False {
                      }
                      frame True {
                        n3607 = call "waveformparamsv2.vi"("command"="rem AO", "index"=w459) -> ()  [unwired: 3 in, 3 out]
                      }
                    }
                  }
                  frame #5 {
                    n3608 = local read "remAO"() -> (w462:bool)
                    n3609 = case shown="True" w462 {
                      tunnel: w461 -> [_ w481]
                      frame False {
                      }
                      frame True {
                        n3610 = local read "Meastab"() -> (w466:enum32{"X-Y Image", "Linescan", "Timetrace"})
                        n3611 = property on="refwf" class="Ring (strict)"() -> ("RingText.Text"=w469:string)  [unwired: 2 in, 2 out]
                        n3612 = case shown="\"Timetrace\"" w466 {
                          tunnel: [w482 w483] -> w465
                          frame "X-Y Image", Default {
                            n3613 = local read "Sampling rate"() -> (w482:dbl)
                          }
                          frame "Timetrace" {
                            n3614 = local read "srateAODOtt"() -> (w483:dbl)
                          }
                        }
                        n3615 = call "waveformsAObuffer.vi"("command"="get") -> ("AO wf out"=w478:waveform(dbl)[])  [unwired: 1 in]
                        n3616 = call "waveformsDObuffer.vi"("command"="get") -> ("DO wf out"=w475:digitalwaveform[])  [unwired: 1 in]
                        n3617 = Delete From Array(array=w478, length=1, index=w481) -> (array with subset deleted=w470:waveform(dbl)[])  [unwired: 1 out]
                        n3618 = call "correctwaveformsizetemp.vi"("new sampling frequency (Hz)"=w465, "start"=FALSE, "reference waveforms to"=w469, "Analog waveforms in"=w470, "stop"=FALSE, "Digital waveforms in"=w475) -> ("analog wf out"=w473:waveform(dbl)[], "Digital wf out"=w471:digitalwaveform[], "measpoints"=w467:i32)
                        n3619 = local write "Analog Lines Plot"(w473) -> ()
                        n3620 = call "GetNumCamFramesv2.vi"("Digital Waveform Graph"=w471) -> ("Numeric"=w472:i32)  [unwired: 10 in]
                        n3621 = local write "Digital Lines Plot"(w471) -> ()
                        n3622 = call "waveformsAObuffer.vi"("AO wf in"=w473, "command"="set") -> ()  [unwired: 1 out]
                        n3623 = call "waveformsDObuffer.vi"("DO wf in"=w471, "command"="set") -> ()  [unwired: 1 out]
                        n3624 = local read "wavdet"() -> (w468:bool)
                        n3625 = local write "Total Camera Frames"(w472) -> ()
                        n3626 = case shown="True" w468 {
                          tunnel: w467 -> [_ w484]
                          frame False {
                          }
                          frame True {
                            n3627 = local write "# of frames"(w484) -> ()
                          }
                        }
                      }
                    }
                  }
                  frame #6 {
                    w485 = FALSE ("remAO")
                    n3628 = local read "finite samples"() -> (w486:bool)
                    n3629 = local read "continuous"() -> (w487:bool)
                    n3630 = local read "wavdet"() -> (w488:bool)
                    n3631 = call "2pparameters.vi"("command"="get") -> ("params out"=w491:T10)  [unwired: 1 in]
                    n3632 = Bundle By Name(cluster=w491, "finite"=w486, "cont"=w487, "wavdet"=w488) -> (w489:T10)
